vi "ConfigureRobot.vi"(3 "Pigeon Ref In":T1={"DeviceStatus"={"status"=FALSE, "code"=0, "source"=""}, "Device Number"=0, "Type"=352321536, "Device ID"=0, "Handle"=0, "UsageFrame"=0, "Library Path"=path ""} {"Type" items=["CAN"=352321536, "TalonSRX"=33554432]}, 4 "Right Side":T3, 5 "Left Side":T3) -> (0 "Pigeon Ref Out":T1={"DeviceStatus"={"status"=FALSE, "code"=0, "source"=""}, "Device Number"=0, "Type"=352321536, "Device ID"=0, "Handle"=0, "UsageFrame"=0, "Library Path"=path ""} {"Type" items=["CAN"=352321536, "TalonSRX"=33554432]}, 1 "Right Side":T3, 2 "Left Side":T3)   [LabVIEW 2018]
uses:
  <vilib>/Rock Robotics/WPI/MotorControl/WPI_MotorControlDeviceRef.ctl
  <vilib>/Rock Robotics/WPI/MotorControl/WPI_MotorControlType.ctl
  <vilib>/Rock Robotics/SystemInterfaces/DIO/FPGA_DIOPWMChannel.ctl
  <vilib>/Rock Robotics/WPI/PWM/WPI_PWMDeadband.ctl
  <vilib>/Rock Robotics/SystemInterfaces/DIO/FPGA_DIOChannel.ctl
  <vilib>/Rock Robotics/WPI/ThirdParty/Phoenix-LabVIEW/Pigeon IMU/CTRE_PigeonIMU_DeviceRef.ctl
  <vilib>/Rock Robotics/WPI/ThirdParty/Phoenix-LabVIEW/Pigeon IMU/CTRE_PigeonIMU_ConnectionType.ctl
  <vilib>/Rock Robotics/WPI/ThirdParty/Phoenix-LabVIEW/Motor Controller/Controls/CTRE_Phoenix_MotorControl_RemoteSourceType.ctl
  <vilib>/Rock Robotics/WPI/ThirdParty/Phoenix-LabVIEW/Motor Controller/Controls/CTRE_Phoenix_MotorControl_SensorTermFeedbackDevice_Enhanced.ctl
  <vilib>/Rock Robotics/WPI/ThirdParty/Phoenix-LabVIEW/Motor Controller/Controls/CTRE_Phoenix_MotorControl_FeedbackDevice.ctl
  <vilib>/Rock Robotics/WPI/ThirdParty/Phoenix-LabVIEW/Motor Controller/Controls/CTRE_Phoenix_MotorControl_StatusFrameEnhanced.ctl
  <vilib>/Rock Robotics/WPI/ThirdParty/Phoenix-LabVIEW/Motor Controller/Controls/CTRE_Phoenix_MotorControl_NeutralMode.ctl
  <vilib>/Rock Robotics/WPI/ThirdParty/Phoenix-LabVIEW/Motor Controller/Controls/CTRE_Phoenix_MotorControl_ControlMode.ctl
  Motor Constants.vi
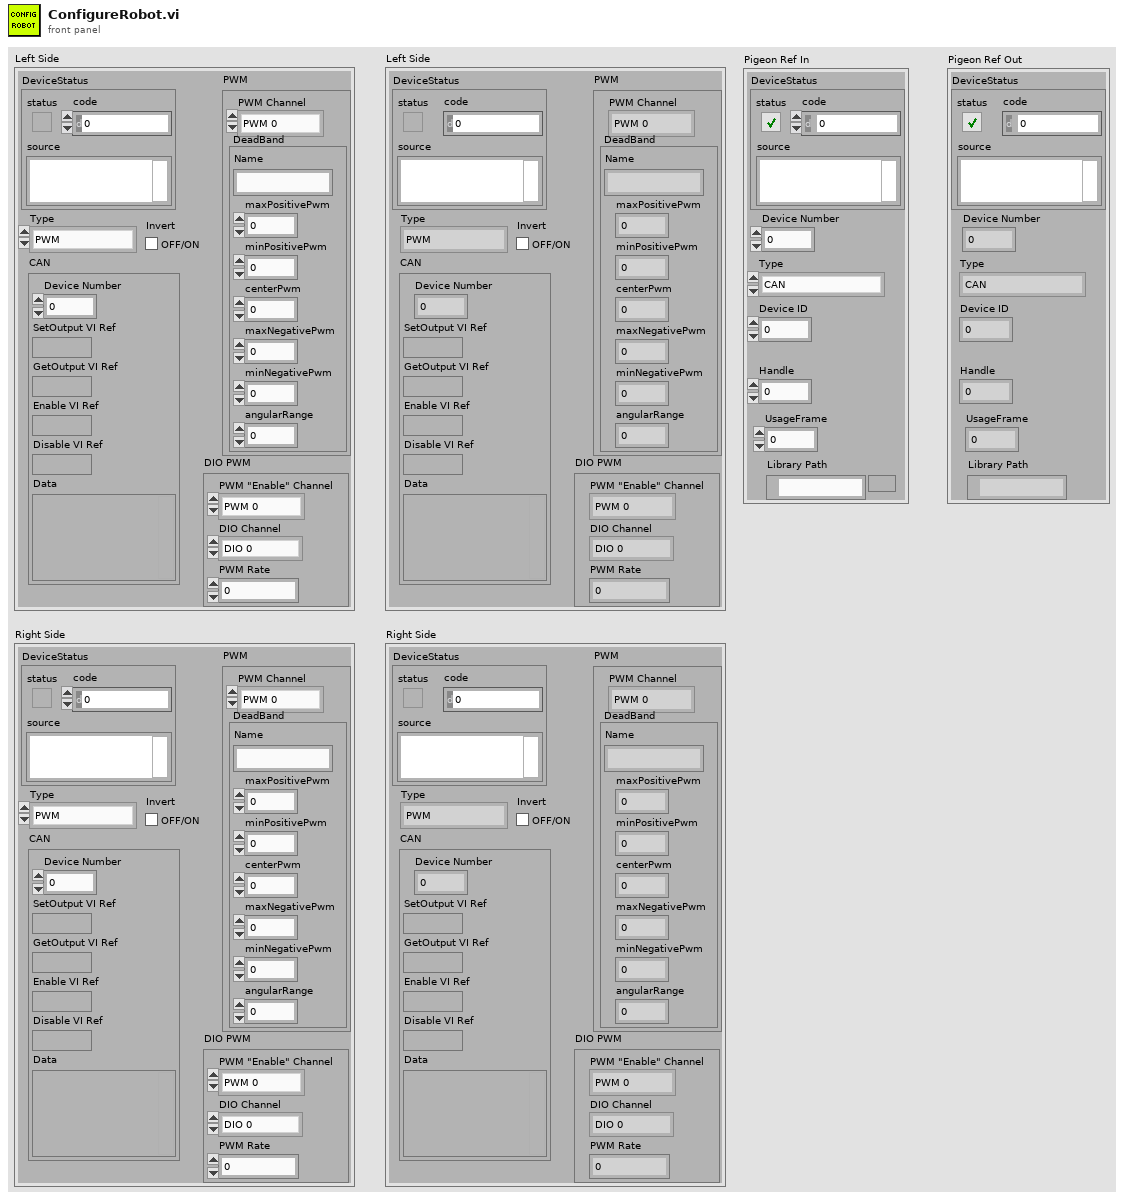
[diagram p1: front panel]
types:
  T1 = typedef "CTRE_PigeonIMU_DeviceRef.ctl" = cluster{"DeviceStatus":errorcluster, "Device Number":u8, "Type":T2, "Device ID":u32, "Handle":u64, "UsageFrame":u32, "Library Path":path}
  T2 = typedef "CTRE_PigeonIMU_ConnectionType.ctl" = u32
  T3 = typedef "WPI_MotorControlDeviceRef.ctl" = cluster{"DeviceStatus":errorcluster, "Type":T4, "PWM":cluster{"PWM Channel":T5, "DeadBand":T6}, "CAN":cluster{"Device Number":u8, "SetOutput VI Ref":variant, "GetOutput VI Ref":variant, "Enable VI Ref":variant, "Disable VI Ref":variant, "Data":variant}, "Invert":bool, "DIO PWM":cluster{"PWM \"Enable\" Channel":T5, "DIOChannel":T7, "PWM Rate":dbl}}
  T4 = typedef "WPI_MotorControlType.ctl" = enum16{"PWM", "CAN", "DIO PWM"}
  T5 = typedef "FPGA_DIOPWMChannel.ctl" = enum8{"PWM 0", "PWM 1", "PWM 2", "PWM 3", "PWM 4", "PWM 5", "PWM 6", "PWM 7", "PWM 8", "PWM 9", "PWM MXP 0", "PWM MXP 1", "PWM MXP 2", "PWM MXP 3", "PWM MXP 4", "PWM MXP 5", "PWM MXP 6", "PWM MXP 7", "PWM MXP 8", "PWM MXP 9", "Invalid"}
  T6 = typedef "WPI_PWMDeadband.ctl" = cluster{"Name":string, "maxPositivePwm":i32, "minPositivePwm":i32, "centerPwm":i32, "maxNegativePwm":i32, "minNegativePwm":i32, "angularRange":u16}
  T7 = typedef "FPGA_DIOChannel.ctl" = enum8{"DIO 0", "DIO 1", "DIO 2", "DIO 3", "DIO 4", "DIO 5", "DIO 6", "DIO 7", "DIO 8", "DIO 9", "DIO MXP 0", "DIO MXP 1", "DIO MXP 2", "DIO MXP 3", "DIO MXP 4", "DIO MXP 5", "DIO MXP 6", "DIO MXP 7", "DIO MXP 8", "DIO MXP 9", "DIO MXP 10", "DIO MXP 11", "DIO MXP 12", "DIO MXP 13", "DIO MXP 14", "DIO MXP 15", "SPI Port CS1", "SPI Port CS2", "SPI Port CS3", "SPI Port MISO", "SPI Port MOSI", "Invalid"}
  T8 = typedef "CTRE_Phoenix_MotorControl_ControlMode.ctl" = u16
  T9 = typedef "CTRE_Phoenix_MotorControl_StatusFrameEnhanced.ctl" = u16
  T10 = typedef "CTRE_Phoenix_MotorControl_FeedbackDevice.ctl" = i8
  T11 = typedef "CTRE_Phoenix_MotorControl_RemoteSourceType.ctl" = enum16{"Off", "Talon SRX Selected Sensor", "Pigeon IMU Yaw", "Pigeon IMU Pitch", "Pigeon IMU Roll", "CANifier Quadrature", "CANifier PWM Input 0", "CANifier PWM Input 1", "CANifier PWM Input 2", "CANifier PWM Input 3", "Gadgeteer Pigeon Yaw", "Gadgeteer Pigeon Pitch", "Gadgeteer Pigeon Roll"}
  T12 = typedef "CTRE_Phoenix_MotorControl_SensorTermFeedbackDevice_Enhanced.ctl" = i8
  T13 = typedef "CTRE_Phoenix_MotorControl_NeutralMode.ctl" = enum8{"EEPROMSetting", "Override to Coast", "Override to Brake"}
  T14 = cluster{"kP":dbl, "kI ":dbl, "kD":dbl, "kF":dbl, "I Zone":dbl, "Peak Out":dbl}
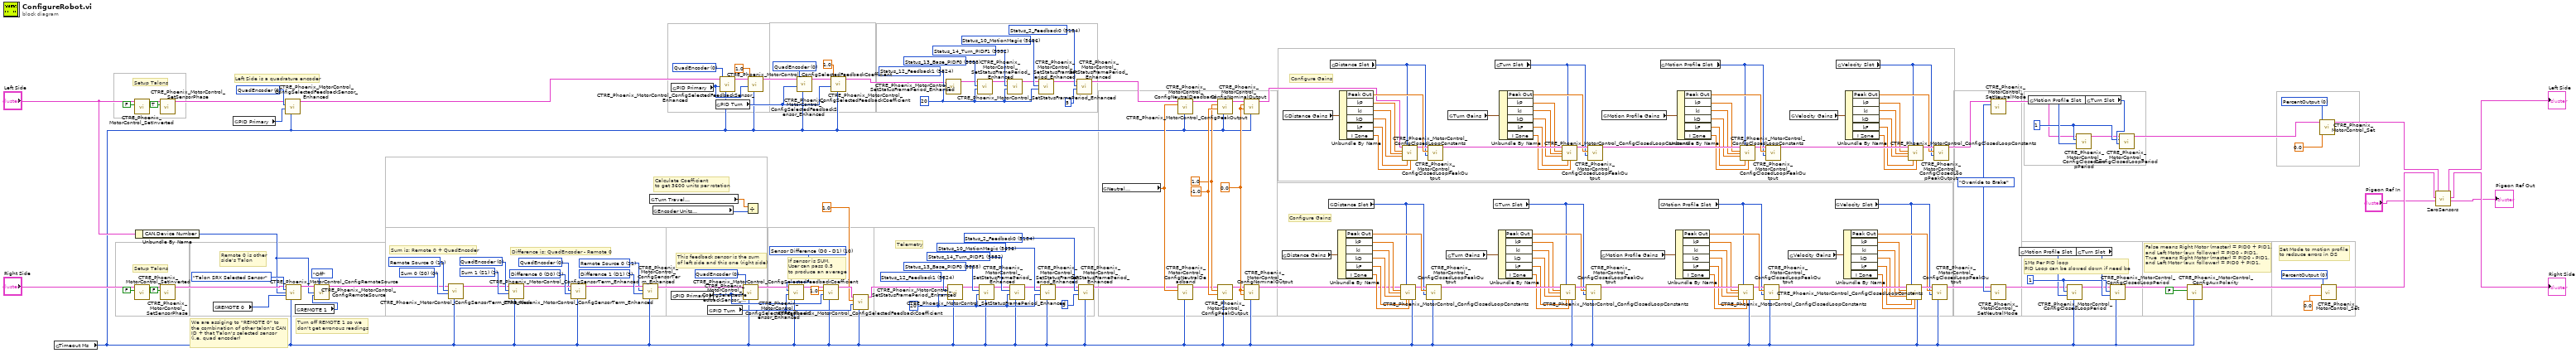
[diagram p0: block diagram]
diagram:
  w6 = T8 0 items=["PercentOutput"=0, "Position"=1, "Velocity"=2, "Current"=3, "Follower"=5, "MotionProfile"=6, "MotionMagic"=7, "MotionProfileArc"=10, "Disabled"=15] ("Control Mode")
  w9 = 1 ("loopTimeMs")
  w64 = T9 5184 items=["Status_1_General"=5120, "Status_2_Feedback0"=5184, "Status_3_Quadrature"=5248, "Status_4_AinTempVbat"=5312, "Status_6_Misc"=5440, "Status_7_CommStatus"=5504, "Status_8_PulseWidth"=5568, "Status_9_MotProfBuffer"=5632, "Status_10_MotionMagic"=5696, "Status_11_UartGadgeteer"=5760, "Status_12_Feedback1"=5824, "Status_13_Base_PIDF0"=5888, "Status_14_Turn_PIDF1"=5952, "Status_15_FirmwareApiStatus"=6016] ("Status Frame")
  w63 = T9 5696 items=["Status_1_General"=5120, "Status_2_Feedback0"=5184, "Status_3_Quadrature"=5248, "Status_4_AinTempVbat"=5312, "Status_6_Misc"=5440, "Status_7_CommStatus"=5504, "Status_8_PulseWidth"=5568, "Status_9_MotProfBuffer"=5632, "Status_10_MotionMagic"=5696, "Status_11_UartGadgeteer"=5760, "Status_12_Feedback1"=5824, "Status_13_Base_PIDF0"=5888, "Status_14_Turn_PIDF1"=5952, "Status_15_FirmwareApiStatus"=6016] ("Status Frame")
  w62 = T9 5952 items=["Status_1_General"=5120, "Status_2_Feedback0"=5184, "Status_3_Quadrature"=5248, "Status_4_AinTempVbat"=5312, "Status_6_Misc"=5440, "Status_7_CommStatus"=5504, "Status_8_PulseWidth"=5568, "Status_9_MotProfBuffer"=5632, "Status_10_MotionMagic"=5696, "Status_11_UartGadgeteer"=5760, "Status_12_Feedback1"=5824, "Status_13_Base_PIDF0"=5888, "Status_14_Turn_PIDF1"=5952, "Status_15_FirmwareApiStatus"=6016] ("Status Frame")
  w61 = T9 5888 items=["Status_1_General"=5120, "Status_2_Feedback0"=5184, "Status_3_Quadrature"=5248, "Status_4_AinTempVbat"=5312, "Status_6_Misc"=5440, "Status_7_CommStatus"=5504, "Status_8_PulseWidth"=5568, "Status_9_MotProfBuffer"=5632, "Status_10_MotionMagic"=5696, "Status_11_UartGadgeteer"=5760, "Status_12_Feedback1"=5824, "Status_13_Base_PIDF0"=5888, "Status_14_Turn_PIDF1"=5952, "Status_15_FirmwareApiStatus"=6016] ("Status Frame")
  w65 = T9 5824 items=["Status_1_General"=5120, "Status_2_Feedback0"=5184, "Status_3_Quadrature"=5248, "Status_4_AinTempVbat"=5312, "Status_6_Misc"=5440, "Status_7_CommStatus"=5504, "Status_8_PulseWidth"=5568, "Status_9_MotProfBuffer"=5632, "Status_10_MotionMagic"=5696, "Status_11_UartGadgeteer"=5760, "Status_12_Feedback1"=5824, "Status_13_Base_PIDF0"=5888, "Status_14_Turn_PIDF1"=5952, "Status_15_FirmwareApiStatus"=6016] ("Status Frame")
  w67 = 20 ("periodMs")
  w68 = T10 0 items=["QuadEncoder"=0, "Analog"=2, "Tachometer"=4, "Pulse Width Encoded Position"=8, "Sensor Sum (S0 + S1)"=9, "Sensor Difference (D0 - D1)"=10, "Remote Source 0"=11, "Remote Source 1"=12, "Software Emulated"=15] ("Feedback Device")
  w69 = T10 0 items=["QuadEncoder"=0, "Analog"=2, "Tachometer"=4, "Pulse Width Encoded Position"=8, "Sensor Sum (S0 + S1)"=9, "Sensor Difference (D0 - D1)"=10, "Remote Source 0"=11, "Remote Source 1"=12, "Software Emulated"=15] ("Feedback Device")
  w89 = T12 0 items=["None"=-1, "QuadEncoder"=0, "Analog"=2, "Tachometer"=4, "Pulse Width Encoded Position"=8, "Remote Source 0"=11, "Remote Source 1"=12, "Software Emulated"=15] ("Feedback Device")
  w90 = T12 11 items=["None"=-1, "QuadEncoder"=0, "Analog"=2, "Tachometer"=4, "Pulse Width Encoded Position"=8, "Remote Source 0"=11, "Remote Source 1"=12, "Software Emulated"=15] ("Feedback Device")
  w97 = T8 0 items=["PercentOutput"=0, "Position"=1, "Velocity"=2, "Current"=3, "Follower"=5, "MotionProfile"=6, "MotionMagic"=7, "MotionProfileArc"=10, "Disabled"=15] ("Control Mode")
  w192 = 1 ("loopTimeMs")
  w188 = CTRE_Phoenix_MotorControl_NeutralMode."Override to Brake" ("Motor Control Neutral Mode")
  w150 = 0.0 ("Forward Nominal Percent Output")
  w147 = -1.0 ("Reverse Peak Percent Output")
  w146 = 1.0 ("Forward Peak Percent Output")
  w93 = 20 ("periodMs")
  w140 = T9 5184 items=["Status_1_General"=5120, "Status_2_Feedback0"=5184, "Status_3_Quadrature"=5248, "Status_4_AinTempVbat"=5312, "Status_6_Misc"=5440, "Status_7_CommStatus"=5504, "Status_8_PulseWidth"=5568, "Status_9_MotProfBuffer"=5632, "Status_10_MotionMagic"=5696, "Status_11_UartGadgeteer"=5760, "Status_12_Feedback1"=5824, "Status_13_Base_PIDF0"=5888, "Status_14_Turn_PIDF1"=5952, "Status_15_FirmwareApiStatus"=6016] ("Status Frame")
  w139 = T9 5696 items=["Status_1_General"=5120, "Status_2_Feedback0"=5184, "Status_3_Quadrature"=5248, "Status_4_AinTempVbat"=5312, "Status_6_Misc"=5440, "Status_7_CommStatus"=5504, "Status_8_PulseWidth"=5568, "Status_9_MotProfBuffer"=5632, "Status_10_MotionMagic"=5696, "Status_11_UartGadgeteer"=5760, "Status_12_Feedback1"=5824, "Status_13_Base_PIDF0"=5888, "Status_14_Turn_PIDF1"=5952, "Status_15_FirmwareApiStatus"=6016] ("Status Frame")
  w138 = T9 5952 items=["Status_1_General"=5120, "Status_2_Feedback0"=5184, "Status_3_Quadrature"=5248, "Status_4_AinTempVbat"=5312, "Status_6_Misc"=5440, "Status_7_CommStatus"=5504, "Status_8_PulseWidth"=5568, "Status_9_MotProfBuffer"=5632, "Status_10_MotionMagic"=5696, "Status_11_UartGadgeteer"=5760, "Status_12_Feedback1"=5824, "Status_13_Base_PIDF0"=5888, "Status_14_Turn_PIDF1"=5952, "Status_15_FirmwareApiStatus"=6016] ("Status Frame")
  w137 = T9 5888 items=["Status_1_General"=5120, "Status_2_Feedback0"=5184, "Status_3_Quadrature"=5248, "Status_4_AinTempVbat"=5312, "Status_6_Misc"=5440, "Status_7_CommStatus"=5504, "Status_8_PulseWidth"=5568, "Status_9_MotProfBuffer"=5632, "Status_10_MotionMagic"=5696, "Status_11_UartGadgeteer"=5760, "Status_12_Feedback1"=5824, "Status_13_Base_PIDF0"=5888, "Status_14_Turn_PIDF1"=5952, "Status_15_FirmwareApiStatus"=6016] ("Status Frame")
  w136 = T9 5824 items=["Status_1_General"=5120, "Status_2_Feedback0"=5184, "Status_3_Quadrature"=5248, "Status_4_AinTempVbat"=5312, "Status_6_Misc"=5440, "Status_7_CommStatus"=5504, "Status_8_PulseWidth"=5568, "Status_9_MotProfBuffer"=5632, "Status_10_MotionMagic"=5696, "Status_11_UartGadgeteer"=5760, "Status_12_Feedback1"=5824, "Status_13_Base_PIDF0"=5888, "Status_14_Turn_PIDF1"=5952, "Status_15_FirmwareApiStatus"=6016] ("Status Frame")
  w88 = T10 10 items=["None"=-1, "QuadEncoder"=0, "Analog"=2, "Tachometer"=4, "Pulse Width Encoded Position"=8, "Sensor Sum (S0 + S1)"=9, "Sensor Difference (D0 - D1)"=10, "Remote Source 0"=11, "Remote Source 1"=12, "Software Emulated"=15] ("Feedback Device")
  w126 = T10 0 items=["None"=-1, "QuadEncoder"=0, "Analog"=2, "Tachometer"=4, "Pulse Width Encoded Position"=8, "Sensor Sum (S0 + S1)"=9, "Sensor Difference (D0 - D1)"=10, "Remote Source 0"=11, "Remote Source 1"=12, "Software Emulated"=15] ("Feedback Device")
  w124 = u16 3 items=["Sum 0 (S0)", "Sum 1 (S1)", "Difference 0 (D0)", "Difference 1 (D1)"] ("Sensor Term")
  w123 = u16 2 items=["Sum 0 (S0)", "Sum 1 (S1)", "Difference 0 (D0)", "Difference 1 (D1)"] ("Sensor Term")
  w118 = u16 1 items=["Sum 0 (S0)", "Sum 1 (S1)", "Difference 0 (D0)", "Difference 1 (D1)"] ("Sensor Term")
  w122 = T12 0 items=["None"=-1, "QuadEncoder"=0, "Analog"=2, "Tachometer"=4, "Pulse Width Encoded Position"=8, "Remote Source 0"=11, "Remote Source 1"=12, "Software Emulated"=15] ("Feedback Device")
  w116 = u16 0 items=["Sum 0 (S0)", "Sum 1 (S1)", "Difference 0 (D0)", "Difference 1 (D1)"] ("Sensor Term")
  w121 = T12 11 items=["None"=-1, "QuadEncoder"=0, "Analog"=2, "Tachometer"=4, "Pulse Width Encoded Position"=8, "Remote Source 0"=11, "Remote Source 1"=12, "Software Emulated"=15] ("Feedback Device")
  w111 = T10 0 items=["None"=-1, "QuadEncoder"=0, "Analog"=2, "Tachometer"=4, "Pulse Width Encoded Position"=8, "Sensor Sum (S0 + S1)"=9, "Sensor Difference (D0 - D1)"=10, "Remote Source 0"=11, "Remote Source 1"=12, "Software Emulated"=15] ("Feedback Device")
  # "Configure Gains"
  # "Turn off REMOTE 1 so we\ndon't get erronous readings"
  # "We are assiging to \"REMOTE 0\" to\nthe combination of other talon's CAN\nID + that Talon's selected sensor\n(i.e. quad encoder)"
  # "Set Mode to motion profile\nto redsuce errors in DS"
  # "False means Right Motor (master) = PID0 + PID1, \nand Left Motor (aux follower) = PID0 - PID1.\nTrue  means Right Motor (master) = PID0 - PID1, \nand Left Motor (aux follower) = PID0 + PID1."
  # "1Ms Per PID loop\nPID Loop can be slowed down if need be"
  # "Configure Gains"
  # "Setup Talons"
  # "Telemetry"
  # "If sensor is SUM,\nUser can pass 0.5\nto produce an average"
  # "Calculate Coefficient\nto get 3600 units per rotation"
  # "This feedback sensor is the sum\nof left side and this one (right side)"
  # "Difference is: QuadEncoder - Remote 0"
  # "Sum is: Remote 0 + QuadEncoder"
  # "Remote 0 is other\nside's Talon"
  # "Left Side is a quadrature encoder"
  # "Setup Talons"
  n1 = global read "Motor Constants.vi" "Timeout Ms"() -> (w70:i32)
  n2 = call <vilib>:"CTRE_Phoenix_MotorControl_SetInverted.vi"("Invert?"=FALSE, "PhoenixMotorControlDevRef"="Left Side") -> ("PhoenixMotorControlDevRef"=w106:T3)  [unwired: 8 in, 1 out]
  n3 = call <vilib>:"CTRE_Phoenix_MotorControl_SetInverted.vi"("Invert?"=FALSE, "PhoenixMotorControlDevRef"="Right Side") -> ("PhoenixMotorControlDevRef"=w107:T3)  [unwired: 8 in, 1 out]
  n4 = Unbundle By Name("Left Side") -> ("CAN.Device Number"=w82:u8)
  n5 = call <vilib>:"CTRE_Phoenix_MotorControl_SetSensorPhase.vi"("PhaseSensor"=TRUE, "PhoenixMotorControlDevRef"=w106) -> ("PhoenixMotorControlDevRef"=w110:T3)  [unwired: 8 in, 1 out]
  n6 = call <vilib>:"CTRE_Phoenix_MotorControl_SetSensorPhase.vi"("PhaseSensor"=FALSE, "PhoenixMotorControlDevRef"=w107) -> ("PhoenixMotorControlDevRef"=w112:T3)  [unwired: 8 in, 1 out]
  n7 = global read "Motor Constants.vi" "REMOTE 0"() -> (w115:i32)
  n8 = global read "Motor Constants.vi" "PID Primary"() -> (w194:i32)
  n9 = call <vilib>:"CTRE_Phoenix_MotorControl_ConfigSelectedFeedbackSensor_Enhanced.vi"("timeoutMs"=w70, "pidLoopIdx"=w194, "Feedback Device"=w111, "PhoenixMotorControlDevRef"=w110) -> ("PhoenixMotorControlDevRef"=w60:T3)  [unwired: 6 in, 1 out]
  n10 = call <vilib>:"CTRE_Phoenix_MotorControl_ConfigRemoteSource.vi"("PhoenixMotorControlDevRef"=w112, "Remote Device Type"=CTRE_Phoenix_MotorControl_RemoteSourceType."Talon SRX Selected Sensor", "Remote Device ID"=w82, "Source Index (0/1)"=w115, "timeoutMs"=w70) -> ("PhoenixMotorControlDevRef"=w85:T3)  [unwired: 9 in, 1 out]
  n11 = global read "Motor Constants.vi" "REMOTE 1"() -> (w83:i32)
  n12 = call <vilib>:"CTRE_Phoenix_MotorControl_ConfigRemoteSource.vi"("PhoenixMotorControlDevRef"=w85, "Remote Device Type"=CTRE_Phoenix_MotorControl_RemoteSourceType."Off", "Remote Device ID"=w82, "Source Index (0/1)"=w83) -> ("PhoenixMotorControlDevRef"=w84:T3)  [unwired: 10 in, 1 out]
  n13 = call <vilib>:"CTRE_Phoenix_MotorControl_ConfigSensorTerm_Enhanced.vi"("timeoutMs"=w70, "Sensor Term"=w116, "Feedback Device"=w121, "PhoenixMotorControlDevRef"=w84) -> ("PhoenixMotorControlDevRef"=w117:T3)  [unwired: 6 in, 1 out]
  n14 = call <vilib>:"CTRE_Phoenix_MotorControl_ConfigSensorTerm_Enhanced.vi"("timeoutMs"=w70, "Sensor Term"=w118, "Feedback Device"=w122, "PhoenixMotorControlDevRef"=w117) -> ("PhoenixMotorControlDevRef"=w120:T3)  [unwired: 6 in, 1 out]
  n15 = call <vilib>:"CTRE_Phoenix_MotorControl_ConfigSensorTerm_Enhanced.vi"("timeoutMs"=w70, "Sensor Term"=w123, "Feedback Device"=w89, "PhoenixMotorControlDevRef"=w120) -> ("PhoenixMotorControlDevRef"=w119:T3)  [unwired: 6 in, 1 out]
  n16 = call <vilib>:"CTRE_Phoenix_MotorControl_ConfigSensorTerm_Enhanced.vi"("timeoutMs"=w70, "Sensor Term"=w124, "Feedback Device"=w90, "PhoenixMotorControlDevRef"=w119) -> ("PhoenixMotorControlDevRef"=w125:T3)  [unwired: 6 in, 1 out]
  n17 = global read "Motor Constants.vi" "Turn Travel\nUnits Per Rotation"() -> (w131:dbl)
  n18 = global read "Motor Constants.vi" "Encoder Units\nPer Rotation"() -> (w92:i32)
  n19 = global read "Motor Constants.vi" "PID Primary"() -> (w91:i32)
  n20 = global read "Motor Constants.vi" "PID Primary"() -> (w75:i32)
  n21 = global read "Motor Constants.vi" "PID Turn"() -> (w130:i32)
  n22 = global read "Motor Constants.vi" "PID Turn"() -> (w72:i32)
  n23 = call <vilib>:"CTRE_Phoenix_MotorControl_ConfigSelectedFeedbackSensor_Enhanced.vi"("timeoutMs"=w70, "pidLoopIdx"=w75, "Feedback Device"=w69, "PhoenixMotorControlDevRef"=w60) -> ("PhoenixMotorControlDevRef"=w76:T3)  [unwired: 6 in, 1 out]
  n24 = call <vilib>:"CTRE_Phoenix_MotorControl_ConfigSelectedFeedbackSensor_Enhanced.vi"("timeoutMs"=w70, "pidLoopIdx"=w91, "Feedback Device"=w126, "PhoenixMotorControlDevRef"=w125) -> ("PhoenixMotorControlDevRef"=w127:T3)  [unwired: 6 in, 1 out]
  n25 = Divide(x=w131, y=w92) -> ()  [unwired: 1 out]
  n26 = call <vilib>:"CTRE_Phoenix_MotorControl_ConfigSelectedFeedbackCoefficient.vi"("timoutMs"=w70, "pidIdx"=w75, "coefficient"=1.0, "PhoenixMotorControlDevRef"=w76) -> ("PhoenixMotorControlDevRef"=w59:T3)  [unwired: 6 in, 1 out]
  n27 = call <vilib>:"CTRE_Phoenix_MotorControl_ConfigSelectedFeedbackSensor_Enhanced.vi"("timeoutMs"=w70, "pidLoopIdx"=w130, "Feedback Device"=w88, "PhoenixMotorControlDevRef"=w127) -> ("PhoenixMotorControlDevRef"=w128:T3)  [unwired: 6 in, 1 out]
  n28 = call <vilib>:"CTRE_Phoenix_MotorControl_ConfigSelectedFeedbackSensor_Enhanced.vi"("timeoutMs"=w70, "pidLoopIdx"=w72, "Feedback Device"=w68, "PhoenixMotorControlDevRef"=w59) -> ("PhoenixMotorControlDevRef"=w73:T3)  [unwired: 6 in, 1 out]
  n29 = call <vilib>:"CTRE_Phoenix_MotorControl_ConfigSelectedFeedbackCoefficient.vi"("timoutMs"=w70, "pidIdx"=w91, "coefficient"=1.0, "PhoenixMotorControlDevRef"=w128) -> ("PhoenixMotorControlDevRef"=w87:T3)  [unwired: 6 in, 1 out]
  n30 = call <vilib>:"CTRE_Phoenix_MotorControl_ConfigSelectedFeedbackCoefficient.vi"("timoutMs"=w70, "pidIdx"=w72, "coefficient"=1.0, "PhoenixMotorControlDevRef"=w73) -> ("PhoenixMotorControlDevRef"=w58:T3)  [unwired: 6 in, 1 out]
  n31 = call <vilib>:"CTRE_Phoenix_MotorControl_ConfigSelectedFeedbackCoefficient.vi"("timoutMs"=w70, "pidIdx"=w130, "coefficient"=1.0, "PhoenixMotorControlDevRef"=w87) -> ("PhoenixMotorControlDevRef"=w86:T3)  [unwired: 6 in, 1 out]
  n32 = call <vilib>:"CTRE_Phoenix_MotorControl_SetStatusFramePeriod_Enhanced.vi"("periodMs"=w67, "Status Frame"=w65, "PhoenixMotorControlDevRef"=w58) -> ("PhoenixMotorControlDevRef"=w57:T3)  [unwired: 7 in, 1 out]
  n33 = call <vilib>:"CTRE_Phoenix_MotorControl_SetStatusFramePeriod_Enhanced.vi"("timeoutMs"=w70, "periodMs"=w93, "Status Frame"=w136, "PhoenixMotorControlDevRef"=w86) -> ("PhoenixMotorControlDevRef"=w132:T3)  [unwired: 6 in, 1 out]
  n34 = call <vilib>:"CTRE_Phoenix_MotorControl_SetStatusFramePeriod_Enhanced.vi"("periodMs"=w67, "Status Frame"=w61, "PhoenixMotorControlDevRef"=w57) -> ("PhoenixMotorControlDevRef"=w56:T3)  [unwired: 7 in, 1 out]
  n35 = call <vilib>:"CTRE_Phoenix_MotorControl_SetStatusFramePeriod_Enhanced.vi"("timeoutMs"=w70, "periodMs"=w93, "Status Frame"=w137, "PhoenixMotorControlDevRef"=w132) -> ("PhoenixMotorControlDevRef"=w133:T3)  [unwired: 6 in, 1 out]
  n36 = call <vilib>:"CTRE_Phoenix_MotorControl_SetStatusFramePeriod_Enhanced.vi"("periodMs"=w67, "Status Frame"=w62, "PhoenixMotorControlDevRef"=w56) -> ("PhoenixMotorControlDevRef"=w55:T3)  [unwired: 7 in, 1 out]
  n37 = call <vilib>:"CTRE_Phoenix_MotorControl_SetStatusFramePeriod_Enhanced.vi"("timeoutMs"=w70, "periodMs"=w93, "Status Frame"=w138, "PhoenixMotorControlDevRef"=w133) -> ("PhoenixMotorControlDevRef"=w134:T3)  [unwired: 6 in, 1 out]
  n38 = call <vilib>:"CTRE_Phoenix_MotorControl_SetStatusFramePeriod_Enhanced.vi"("periodMs"=w67, "Status Frame"=w63, "PhoenixMotorControlDevRef"=w55) -> ("PhoenixMotorControlDevRef"=w54:T3)  [unwired: 7 in, 1 out]
  n39 = call <vilib>:"CTRE_Phoenix_MotorControl_SetStatusFramePeriod_Enhanced.vi"("timeoutMs"=w70, "periodMs"=w93, "Status Frame"=w139, "PhoenixMotorControlDevRef"=w134) -> ("PhoenixMotorControlDevRef"=w135:T3)  [unwired: 6 in, 1 out]
  n40 = call <vilib>:"CTRE_Phoenix_MotorControl_SetStatusFramePeriod_Enhanced.vi"("periodMs"=5, "Status Frame"=w64, "PhoenixMotorControlDevRef"=w54) -> ("PhoenixMotorControlDevRef"=w53:T3)  [unwired: 7 in, 1 out]
  n41 = call <vilib>:"CTRE_Phoenix_MotorControl_SetStatusFramePeriod_Enhanced.vi"("timeoutMs"=w70, "periodMs"=5, "Status Frame"=w140, "PhoenixMotorControlDevRef"=w135) -> ("PhoenixMotorControlDevRef"=w142:T3)  [unwired: 6 in, 1 out]
  n42 = global read "Motor Constants.vi" "Neutral\nDeadband"() -> (w144:dbl)
  n43 = call <vilib>:"CTRE_Phoenix_MotorControl_ConfigNeutralDeadband.vi"("timeoutMs"=w70, "Percent Deadband"=w144, "PhoenixMotorControlDevRef"=w53) -> ("PhoenixMotorControlDevRef"=w145:T3)  [unwired: 7 in, 1 out]
  n44 = call <vilib>:"CTRE_Phoenix_MotorControl_ConfigNeutralDeadband.vi"("timeoutMs"=w70, "Percent Deadband"=w144, "PhoenixMotorControlDevRef"=w142) -> ("PhoenixMotorControlDevRef"=w143:T3)  [unwired: 7 in, 1 out]
  n45 = call <vilib>:"CTRE_Phoenix_MotorControl_ConfigPeakOutput.vi"("timeoutMs"=w70, "Reverse Peak Percent Output"=w147, "Forward Peak Percent Output"=w146, "PhoenixMotorControlDevRef"=w145) -> ("PhoenixMotorControlDevRef"=w149:T3)  [unwired: 6 in, 1 out]
  n46 = call <vilib>:"CTRE_Phoenix_MotorControl_ConfigPeakOutput.vi"("timeoutMs"=w70, "Reverse Peak Percent Output"=w147, "Forward Peak Percent Output"=w146, "PhoenixMotorControlDevRef"=w143) -> ("PhoenixMotorControlDevRef"=w148:T3)  [unwired: 6 in, 1 out]
  n47 = call <vilib>:"CTRE_Phoenix_MotorControl_ConfigNominalOutput.vi"("timeoutMs"=w70, "Reverse Nominal Percent Output"=w150, "Forward Nominal Percent Output"=w150, "PhoenixMotorControlDevRef"=w149) -> ("PhoenixMotorControlDevRef"=w13:T3)  [unwired: 6 in, 1 out]
  n48 = call <vilib>:"CTRE_Phoenix_MotorControl_ConfigNominalOutput.vi"("timeoutMs"=w70, "Reverse Nominal Percent Output"=w150, "Forward Nominal Percent Output"=w150, "PhoenixMotorControlDevRef"=w148) -> ("PhoenixMotorControlDevRef"=w151:T3)  [unwired: 6 in, 1 out]
  n49 = global read "Motor Constants.vi" "Distance Gains"() -> (w152:T14)
  n50 = global read "Motor Constants.vi" "Distance Gains"() -> (w18:T14)
  n51 = global read "Motor Constants.vi" "Distance Slot"() -> (w100:i32)
  n52 = global read "Motor Constants.vi" "Distance Slot"() -> (w16:i32)
  n53 = Unbundle By Name(w152) -> ("Peak Out"=w159:dbl, "kP"=w153:dbl, "kI"=w154:dbl, "kD"=w155:dbl, "kF"=w156:dbl, "I Zone"=w157:dbl)
  n54 = Unbundle By Name(w18) -> ("Peak Out"=w25:dbl, "kP"=w19:dbl, "kI"=w20:dbl, "kD"=w21:dbl, "kF"=w22:dbl, "I Zone"=w23:dbl)
  n55 = call <vilib>:"CTRE_Phoenix_MotorControl_ConfigClosedLoopConstants.vi"("PhoenixMotorControlDevRef"=w151, "slotIdx"=w100, "P"=w153, "I"=w154, "D"=w155, "F"=w156, "I Zone"=w157, "timeoutMs"=w70) -> ("PhoenixMotorControlDevRef"=w158:T3)  [unwired: 6 in, 1 out]
  n56 = call <vilib>:"CTRE_Phoenix_MotorControl_ConfigClosedLoopConstants.vi"("PhoenixMotorControlDevRef"=w13, "slotIdx"=w16, "P"=w19, "I"=w20, "D"=w21, "F"=w22, "I Zone"=w23) -> ("PhoenixMotorControlDevRef"=w24:T3)  [unwired: 7 in, 1 out]
  n57 = call <vilib>:"CTRE_Phoenix_MotorControl_ConfigClosedLoopPeakOutput.vi"("timoutMs"=w70, "slotIdx"=w100, "peakOutput"=w159, "PhoenixMotorControlDevRef"=w158) -> ("PhoenixMotorControlDevRef"=w184:T3)  [unwired: 6 in, 1 out]
  n58 = call <vilib>:"CTRE_Phoenix_MotorControl_ConfigClosedLoopPeakOutput.vi"("slotIdx"=w16, "peakOutput"=w25, "PhoenixMotorControlDevRef"=w24) -> ("PhoenixMotorControlDevRef"=w50:T3)  [unwired: 7 in, 1 out]
  n59 = global read "Motor Constants.vi" "Turn Gains"() -> (w167:T14)
  n60 = global read "Motor Constants.vi" "Turn Gains"() -> (w33:T14)
  n61 = global read "Motor Constants.vi" "Turn Slot"() -> (w99:i32)
  n62 = global read "Motor Constants.vi" "Turn Slot"() -> (w15:i32)
  n63 = Unbundle By Name(w167) -> ("Peak Out"=w160:dbl, "kP"=w166:dbl, "kI"=w165:dbl, "kD"=w164:dbl, "kF"=w163:dbl, "I Zone"=w162:dbl)
  n64 = Unbundle By Name(w33) -> ("Peak Out"=w26:dbl, "kP"=w32:dbl, "kI"=w31:dbl, "kD"=w30:dbl, "kF"=w29:dbl, "I Zone"=w28:dbl)
  n65 = call <vilib>:"CTRE_Phoenix_MotorControl_ConfigClosedLoopConstants.vi"("PhoenixMotorControlDevRef"=w184, "slotIdx"=w99, "P"=w166, "I"=w165, "D"=w164, "F"=w163, "I Zone"=w162, "timeoutMs"=w70) -> ("PhoenixMotorControlDevRef"=w161:T3)  [unwired: 6 in, 1 out]
  n66 = call <vilib>:"CTRE_Phoenix_MotorControl_ConfigClosedLoopConstants.vi"("PhoenixMotorControlDevRef"=w50, "slotIdx"=w15, "P"=w32, "I"=w31, "D"=w30, "F"=w29, "I Zone"=w28) -> ("PhoenixMotorControlDevRef"=w27:T3)  [unwired: 7 in, 1 out]
  n67 = call <vilib>:"CTRE_Phoenix_MotorControl_ConfigClosedLoopPeakOutput.vi"("timoutMs"=w70, "slotIdx"=w99, "peakOutput"=w160, "PhoenixMotorControlDevRef"=w161) -> ("PhoenixMotorControlDevRef"=w185:T3)  [unwired: 6 in, 1 out]
  n68 = call <vilib>:"CTRE_Phoenix_MotorControl_ConfigClosedLoopPeakOutput.vi"("slotIdx"=w15, "peakOutput"=w26, "PhoenixMotorControlDevRef"=w27) -> ("PhoenixMotorControlDevRef"=w51:T3)  [unwired: 7 in, 1 out]
  n69 = global read "Motor Constants.vi" "Motion Profile Gains"() -> (w168:T14)
  n70 = global read "Motor Constants.vi" "Motion Profile Gains"() -> (w34:T14)
  n71 = global read "Motor Constants.vi" "Motion Profile Slot"() -> (w101:i32)
  n72 = global read "Motor Constants.vi" "Motion Profile Slot"() -> (w17:i32)
  n73 = Unbundle By Name(w168) -> ("Peak Out"=w175:dbl, "kP"=w169:dbl, "kI"=w170:dbl, "kD"=w171:dbl, "kF"=w172:dbl, "I Zone"=w173:dbl)
  n74 = Unbundle By Name(w34) -> ("Peak Out"=w41:dbl, "kP"=w35:dbl, "kI"=w36:dbl, "kD"=w37:dbl, "kF"=w38:dbl, "I Zone"=w39:dbl)
  n75 = call <vilib>:"CTRE_Phoenix_MotorControl_ConfigClosedLoopConstants.vi"("PhoenixMotorControlDevRef"=w185, "slotIdx"=w101, "P"=w169, "I"=w170, "D"=w171, "F"=w172, "I Zone"=w173, "timeoutMs"=w70) -> ("PhoenixMotorControlDevRef"=w174:T3)  [unwired: 6 in, 1 out]
  n76 = call <vilib>:"CTRE_Phoenix_MotorControl_ConfigClosedLoopConstants.vi"("PhoenixMotorControlDevRef"=w51, "slotIdx"=w17, "P"=w35, "I"=w36, "D"=w37, "F"=w38, "I Zone"=w39) -> ("PhoenixMotorControlDevRef"=w40:T3)  [unwired: 7 in, 1 out]
  n77 = call <vilib>:"CTRE_Phoenix_MotorControl_ConfigClosedLoopPeakOutput.vi"("timoutMs"=w70, "slotIdx"=w101, "peakOutput"=w175, "PhoenixMotorControlDevRef"=w174) -> ("PhoenixMotorControlDevRef"=w186:T3)  [unwired: 6 in, 1 out]
  n78 = call <vilib>:"CTRE_Phoenix_MotorControl_ConfigClosedLoopPeakOutput.vi"("slotIdx"=w17, "peakOutput"=w41, "PhoenixMotorControlDevRef"=w40) -> ("PhoenixMotorControlDevRef"=w52:T3)  [unwired: 7 in, 1 out]
  n79 = global read "Motor Constants.vi" "Velocity Gains"() -> (w183:T14)
  n80 = global read "Motor Constants.vi" "Velocity Gains"() -> (w49:T14)
  n81 = global read "Motor Constants.vi" "Velocity Slot"() -> (w98:i32)
  n82 = global read "Motor Constants.vi" "Velocity Slot"() -> (w14:i32)
  n83 = Unbundle By Name(w183) -> ("Peak Out"=w176:dbl, "kP"=w182:dbl, "kI"=w181:dbl, "kD"=w180:dbl, "kF"=w179:dbl, "I Zone"=w178:dbl)
  n84 = Unbundle By Name(w49) -> ("Peak Out"=w42:dbl, "kP"=w48:dbl, "kI"=w47:dbl, "kD"=w46:dbl, "kF"=w45:dbl, "I Zone"=w44:dbl)
  n85 = call <vilib>:"CTRE_Phoenix_MotorControl_ConfigClosedLoopConstants.vi"("PhoenixMotorControlDevRef"=w186, "slotIdx"=w98, "P"=w182, "I"=w181, "D"=w180, "F"=w179, "I Zone"=w178, "timeoutMs"=w70) -> ("PhoenixMotorControlDevRef"=w177:T3)  [unwired: 6 in, 1 out]
  n86 = call <vilib>:"CTRE_Phoenix_MotorControl_ConfigClosedLoopConstants.vi"("PhoenixMotorControlDevRef"=w52, "slotIdx"=w14, "P"=w48, "I"=w47, "D"=w46, "F"=w45, "I Zone"=w44) -> ("PhoenixMotorControlDevRef"=w43:T3)  [unwired: 7 in, 1 out]
  n87 = call <vilib>:"CTRE_Phoenix_MotorControl_ConfigClosedLoopPeakOutput.vi"("timoutMs"=w70, "slotIdx"=w98, "peakOutput"=w176, "PhoenixMotorControlDevRef"=w177) -> ("PhoenixMotorControlDevRef"=w187:T3)  [unwired: 6 in, 1 out]
  n88 = call <vilib>:"CTRE_Phoenix_MotorControl_ConfigClosedLoopPeakOutput.vi"("slotIdx"=w14, "peakOutput"=w42, "PhoenixMotorControlDevRef"=w43) -> ("PhoenixMotorControlDevRef"=w12:T3)  [unwired: 7 in, 1 out]
  n89 = call <vilib>:"CTRE_Phoenix_MotorControl_SetNeutralMode.vi"("Motor Control Neutral Mode"=w188, "PhoenixMotorControlDevRef"=w12) -> ("PhoenixMotorControlDevRef"=w7:T3)  [unwired: 8 in, 1 out]
  n90 = call <vilib>:"CTRE_Phoenix_MotorControl_SetNeutralMode.vi"("Motor Control Neutral Mode"=w188, "PhoenixMotorControlDevRef"=w187) -> ("PhoenixMotorControlDevRef"=w189:T3)  [unwired: 8 in, 1 out]
  n91 = global read "Motor Constants.vi" "Motion Profile Slot"() -> (w190:i32)
  n92 = global read "Motor Constants.vi" "Motion Profile Slot"() -> (w11:i32)
  n93 = call <vilib>:"CTRE_Phoenix_MotorControl_ConfigClosedLoopPeriod.vi"("timoutMs"=w70, "slotIdx"=w190, "loopTimeMs"=w192, "PhoenixMotorControlDevRef"=w189) -> ("PhoenixMotorControlDevRef"=w191:T3)  [unwired: 6 in, 1 out]
  n94 = call <vilib>:"CTRE_Phoenix_MotorControl_ConfigClosedLoopPeriod.vi"("slotIdx"=w11, "loopTimeMs"=w9, "PhoenixMotorControlDevRef"=w7) -> ("PhoenixMotorControlDevRef"=w8:T3)  [unwired: 7 in, 1 out]
  n95 = global read "Motor Constants.vi" "Turn Slot"() -> (w193:i32)
  n96 = global read "Motor Constants.vi" "Turn Slot"() -> (w10:i32)
  n97 = call <vilib>:"CTRE_Phoenix_MotorControl_ConfigClosedLoopPeriod.vi"("timoutMs"=w70, "slotIdx"=w193, "loopTimeMs"=w192, "PhoenixMotorControlDevRef"=w191) -> ("PhoenixMotorControlDevRef"=w103:T3)  [unwired: 6 in, 1 out]
  n98 = call <vilib>:"CTRE_Phoenix_MotorControl_ConfigClosedLoopPeriod.vi"("slotIdx"=w10, "loopTimeMs"=w9, "PhoenixMotorControlDevRef"=w8) -> ("PhoenixMotorControlDevRef"=w4:T3)  [unwired: 7 in, 1 out]
  n99 = call <vilib>:"CTRE_Phoenix_MotorControl_ConfigAuxPolarity.vi"("timeoutMs"=w70, "Invert"=FALSE, "PhoenixMotorControlDevRef"=w103) -> ("PhoenixMotorControlDevRef"=w95:T3)  [unwired: 7 in, 1 out]
  n100 = call <vilib>:"CTRE_Phoenix_MotorControl_Set.vi"("Output"=0.0, "Control Mode"=w6, "PhoenixMotorControlDevRef"=w4) -> ("PhoenixMotorControlDevRef"=w3:T3)  [unwired: 7 in, 1 out]
  n101 = call <vilib>:"CTRE_Phoenix_MotorControl_Set.vi"("Output"=0.0, "Control Mode"=w97, "PhoenixMotorControlDevRef"=w95) -> ("PhoenixMotorControlDevRef"=w80:T3)  [unwired: 7 in, 1 out]
  n102 = call "ZeroSensors.vi"("Pigeon"="Pigeon Ref In", "Talon 2"=w80, "Talon 1"=w3) -> ("Pigeon"=→"Pigeon Ref Out":T1, "Talon 2"=→"Right Side":T3, "Talon 1"=→"Left Side":T3)  [unwired: 6 in]
